vi "ai and ao debug (fpga).vi"() -> ()   [LabVIEW 2019]
uses:
  <vilib>/Platform/TimedLoop/XDataNode/wakeup.ctl
  <vilib>/Platform/TimedLoop/XDataNode/XDNodeRunTimeDep.lvlib
  <vilib>/Platform/TimedLoop/XDataNode/nitl_modes.ctl
  <vilib>/Platform/TimedLoop/XDataNode/timing_clust.ctl
  <vilib>/Platform/TimedLoop/XDataNode/XDataNode.xnode
  <vilib>/eio/EIONode/EIONode.xnode
  <vilib>/rvi/eio/common/nirviEmuTemplateMethod_errors.vi
  Controls/SPI Channels.ctl
  <userlib>/_NI SPI IP/FPGA/Controllers/Public/Spi Master Inputs.ctl
  <vilib>/eio/EIOMethodNode/EIOMethodNode.xnode
  <userlib>/_NI SPI IP/FPGA/Controllers/Public/Transfer Settings.ctl
panel:
  in  "Onboard AI Data In":u64 format="%.0x"
  out "Onboard AI":u16[](array[numeric])
  in  "Onboard AI SPI Settings":T1 {"Direction Change Bit" max=64 step=1; "Transfer Length (bits)" min=1 max=64 step=1}
  out "Onboard AI Data":u64 format="%.0x"
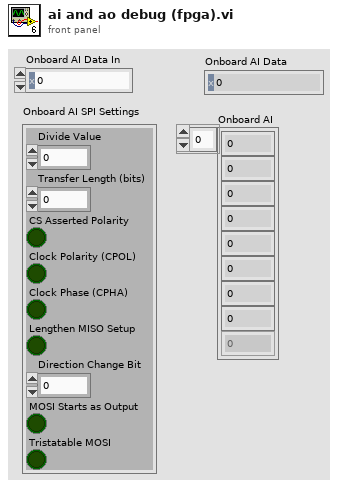
[diagram p1: front panel]
types:
  T1 = typedef "DIO SPI FPGA.lvlib/Transfer Settings.ctl" = cluster{"Divide Value":u8, "Transfer Length (bits)":u8, "CS Asserted Polarity":bool, "Clock Polarity (CPOL)":bool, "Clock Phase (CPHA)":bool, "Lengthen MISO Setup":bool, "Direction Change Bit":u8, "MOSI Starts as Output":bool, "Tristatable MOSI":bool}
  T2 = typedef "SPI Channels.ctl" = cluster{"CS":refnum<k21>, "CLK":refnum<k21>, "MOSI":refnum<k21>, "MISO":refnum<k21>}
  T3 = typedef "XDNodeRunTimeDep.lvlib/timing_clust.ctl" = cluster{"Expected End [f-1]":u64, "Actual End [f-1]":u64, "Finished Late? [f-1]":bool, "Expected End [i-1]":u64, "Actual End [i-1]":u64, "Finished Late? [i-1]":bool, "Expected Start [i]":u64, "Actual Start [i]":u64, "Expected Start [f]":u64, "Actual Start [f]":u64, "Source Name":string, "Structure Name":string, "Period":i64, "Deadline":i64, "Offset":i64, "Start":i64, "Priority":i32, "Timeout":i32, "Mode":T4, "Wakeup Reason":T5, "Error":errorcluster, "Source Type":string, "Secondary Source Type":string, "Global End Time":u64, "Global Start Time":u64, "Frame Duration":u64, "Iteration Duration":u64, "Assigned CPU":i32, "I/O Scan Engine Mode":u32}
  T4 = typedef "XDNodeRunTimeDep.lvlib/nitl_modes.ctl" = enum32{"No Change", "Process missed periods, maintain original phase", "Discard missed periods, maintain original phase", "Process missed periods, ignore original phase", "Discard missed periods, ignore original phase"}
  T5 = typedef "XDNodeRunTimeDep.lvlib/wakeup.ctl" = enum32{"Normal", "Aborted", "Asynchronous wakeup", "Timing source error", "Timed loop error", "Timeout"}
  T6 = typedef "DIO SPI FPGA.lvlib/Spi Master Inputs.ctl" = cluster{"MISO":bool}
  T7 = typedef "DIO SPI FPGA.lvlib/Spi Master Outputs.ctl" = cluster{"Chip Select":bool, "Clock":bool, "MOSI":bool, "MOSI OE":bool}
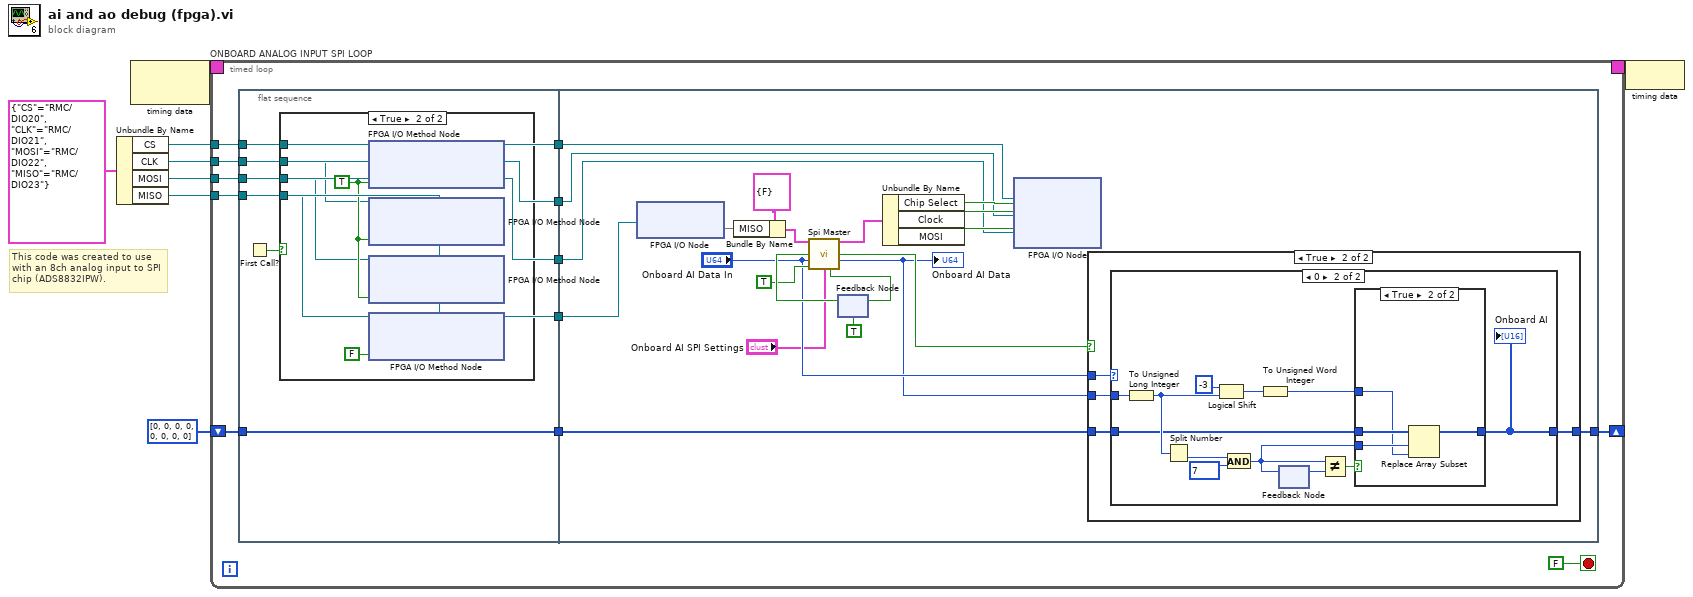
[diagram p0: block diagram]
diagram:
  # "This code was created to use\nwith an 8ch analog input to SPI\nchip (ADS8832IPW)."
  n1 = Unbundle By Name(T2 {"CS"="RMC/DIO20", "CLK"="RMC/DIO21", "MOSI"="RMC/DIO22", "MISO"="RMC/DIO23"} ("SPI Channels")) -> ("CS"=w2:refnum<k21>, "CLK"=w3:refnum<k21>, "MOSI"=w4:refnum<k21>, "MISO"=w5:refnum<k21>)
  n2 = node-c288() -> (w8:T3)  [unwired: 1 in]
  n3 = timed-loop "ONBOARD ANALOG INPUT SPI LOOP" {
    timing: w8 -> [_]
    timing-out: [_] -> w7
    shift-right: [w17] -> _
    shift-left: u16[] [0, 0, 0, 0, 0, 0, 0, 0] -> [w18]
    tunnel: w2 -> [w16]
    tunnel: w3 -> [w15]
    tunnel: w4 -> [w14]
    tunnel: w5 -> [w13]
    stop <- FALSE stop-if-true
    n4 = flat-sequence {
      tunnel: [w25] -> w19
      tunnel: w18 -> [w25]
      tunnel: w16 -> [w24]
      tunnel: w15 -> [w23]
      tunnel: w14 -> [w22]
      tunnel: w13 -> [w21]
      tunnel: [w24] -> w12
      tunnel: [w23] -> w11
      tunnel: [w22] -> w10
      tunnel: [w21] -> w9
      tunnel: w19 -> [w40]
      tunnel: [w39] -> w17
      tunnel: w12 -> [w38]
      tunnel: w11 -> [w37]
      tunnel: w10 -> [w36]
      tunnel: w9 -> [w35]
      frame #0 {
        n5 = First Call?() -> (First Call?: T/F=w26:bool)
        n6 = case shown="True" w26 {
          tunnel: w24 -> [_ w30]
          tunnel: w23 -> [_ w29]
          tunnel: w22 -> [_ w28]
          tunnel: w21 -> [_ w27]
          frame False {
          }
          frame True {
            w32 = TRUE ("Enable")
            n7 = xnode "FPGA I/O Method Node"("FPGA I/O In"=w30, "Enable"=w32) -> ()  [unwired: 1 out]
            n8 = xnode "FPGA I/O Method Node"("FPGA I/O In"=w29, "Enable"=w32) -> ()  [unwired: 1 out]
            n9 = xnode "FPGA I/O Method Node"("FPGA I/O In"=w28, "Enable"=w32) -> ()  [unwired: 1 out]
            n10 = xnode "FPGA I/O Method Node"("FPGA I/O In"=w27, "Enable"=FALSE) -> ()  [unwired: 1 out]
          }
        }
      }
      frame #1 {
        n11 = xnode "FPGA I/O Node"("FPGA I/O In"=w35) -> ("I/O Item"=w47)  [unwired: 1 out]
        n12 = Bundle By Name(cluster=T6 {"MISO"=FALSE} ("spi input"), "MISO"=w47) -> (w48:T6)
        n13 = feedback #1(TRUE ("read data valid")) -> (w45:bool)
        n14 = call <userlib>:"Spi Master.vi"("spi input"=w48, "start strobe"=w45, "data to write"="Onboard AI Data In", "MOSI output enable done"=TRUE, "spi transfer settings"="Onboard AI SPI Settings") -> ("spi output"=w53:T7, "read data valid"=w41:bool, "read data"=w33:u64, "ready for input"=w42:bool)  [unwired: 7 in]
        "Onboard AI Data" <- w33
        n15 = feedback-in #1(w42) -> ()
        n16 = Unbundle By Name(w53) -> ("Chip Select"=w52:bool, "Clock"=w51:bool, "MOSI"=w50:bool)
        n17 = xnode "FPGA I/O Node"("I/O Item"=w52, "FPGA I/O In"=w38, "I/O Item"=w51, "FPGA I/O In"=w37, "I/O Item"=w50, "FPGA I/O In"=w36) -> ()  [unwired: 3 out]
        n18 = case shown="True" w41 {
          tunnel: "Onboard AI Data In" -> [_ w58]
          tunnel: w40 -> [w54 w57]
          tunnel: [w54 w56] -> w39
          tunnel: w33 -> [_ w55]
          frame False {
          }
          frame True {
            n19 = case shown="0" w58 {
              tunnel: w57 -> [w59 w65]
              tunnel: [w59 w64] -> w56
              tunnel: w55 -> [_ w61]
              frame Default {
              }
              frame 0 {
                n20 = To Unsigned Long Integer(number=w61) -> (unsigned 32bit integer=w66:u32)
                n21 = Split Number(x=w66) -> (lo(x)=w70:u16)  [unwired: 1 out]
                n22 = Logical Shift(y=i16 -3, x=w66) -> (x << y=w67:u32)
                n23 = And(x=w70, y=u16 7) -> (x .and. y?=w62:u16)
                n24 = To Unsigned Word Integer(number=w67) -> (unsigned 16bit integer=w60:u16)
                n25 = feedback #2() -> (w71:u16)  [unwired: 1 in]
                n26 = feedback-in #2(w62) -> ()
                n27 = Not Equal?(x=w62, y=w71) -> (x != y?=w63:bool)
                n28 = case shown="True" w63 {
                  tunnel: w65 -> [w72 w76]
                  tunnel: [w72 w75] -> w64
                  tunnel: w62 -> [_ w74]
                  tunnel: w60 -> [_ w73]
                  frame False {
                  }
                  frame True {
                    n29 = Replace Array Subset(array=w76, new element=w73, index=w74) -> (w75:u16[])
                  }
                }
                "Onboard AI" <- w64
              }
            }
          }
        }
      }
    }
  }
  n30 = node-c288(w7) -> ()
